vi "Double FFT Mesurament RT with Frequency Linearization & BackNoise Remove Test.vi"() -> ()   [LabVIEW 2014]
uses:
  <vilib>/Platform/TimedLoop/XDataNode/timing_clust.ctl
  <vilib>/Platform/TimedLoop/XDataNode/nitl_modes.ctl
  <vilib>/Platform/TimedLoop/XDataNode/wakeup.ctl
  <vilib>/FPGAPlugInAG/sbRIO-9636/niLvFpga_Open_sbRIO-9636.vi
  <vilib>/rvi/interface/common/dynamic/niFpgaDynamicAddResources.vi
  <vilib>/FPGAPlugInAG/Dynamic/niLvFpga_Reset_Dynamic.vi
  <vilib>/Utility/error.llb/Error Cluster From Error Code.vi
  <vilib>/rvi/errors/niLvFpgaAdjustHostInterfaceError.vi
  <vilib>/rvi/interface/common/niFpgaWaitOnOcc.vi
  <vilib>/FPGAPlugInAG/Dynamic/niLvFpga_Run_Dynamic.vi
  <vilib>/FPGAPlugInAG/Dynamic/niLvFpga_Abort_Dynamic.vi
  <vilib>/FPGAPlugInAG/Dynamic/niLvFpga_Close_Dynamic.vi
  <vilib>/rvi/interface/nirviOpenFPGA/nirviOpenFPGA.xnode
  FPGA Bitfiles/LaserDistanceSen_FPGATarget_DoubleFFTMesuram_6dDziXQAIGE.lvbitx
  FPGA Target/Test VIs/Double FFT Mesurament Test with Background Noise Remove.vi
  <vilib>/rvi/interface/nirviMethod/nirviMethod.xnode
  <vilib>/rvi/interface/nirviReadWriteControl/nirviReadWriteControl.xnode
  <vilib>/Platform/TimedLoop/XDataNode/XDataNode.xnode
  <vilib>/rvi/interface/nirviCloseFPGA/nirviCloseFPGA.xnode
  <vilib>/FPGAPlugInAG/Dynamic/niLvFpga_ConfigureFifo_Dynamic.vi
  <vilib>/rvi/errors/niLvFpgaMergeErrorWithErrorCode.vi
  <vilib>/FPGAPlugInAG/Dynamic/niLvFpga_StartFifo_Dynamic.vi
  <vilib>/rvi/interface/Simulation/niFpgaSimulationCallBeginRW.vi
  <vilib>/FPGAPlugInAG/Dynamic/niLvFpga_ReadFifo_Dynamic.vi
  <vilib>/Platform/TimedLoop/XDataNode/XDNodeRunTimeDep.lvlib
  NiFpgaLv.dll
panel:
  in  "Active PolyFit":bool
  out "2) Max-Min error":dbl
  out "1) Max-Min error":dbl
  in  "polynomial order":i32=3
  in  "side points":i32=6
  out "2^(n-bit) misure mediate":dbl
  in  "n-bit":i32=10
  in  "SubtractionType":T1(ring)=enum."LowPass"
  out "Fondo Signal":dbl[](graph)
  in  "LowPass Filter: Low cutoff frequency":dbl=1000000.0 format="%#_13g"
  in  "PolyFitting: Poly Grade":dbl=12.0
  in  "Scale Factor Rising":dbl=0.5
  out "2) Std Dev":dbl
  out "1) Std Dev":dbl
  in  "Scale Factor Falling":dbl=0.5
  in  "Triangolo dritto":bool
  in  "Acrive  Smooth":bool
  out "Complete SkewTri":dbl[](graph)
  out "2) Tri edge RISING":dbl[](graph)
  out "1) Tri edge FALLING":dbl[](graph)
  out "1) Ext Mean Time Curve":dbl[](graph)
  out "2) Ext Mean Time Curve":dbl[](graph)
  out "2) Mean Freq Curve Rising":dbl[](graph)
  out "1) Mean Freq Curve Falling":dbl[](graph)
  out "2) Freq curve":dbl[](graph)
  out "1) Freq curve":dbl[](graph)
  in  "FFT Sliding Win Size":i32=128
  out "1) SmoothSubSig":dbl[](graph)
  out "2) SmoothSubSig":dbl[](graph)
  in  "Acrive Fit":bool=TRUE
  in  "Poly Order":i32=3
  in  "Side points":i32=13
  in  "Poly Grade":dbl=5.0
  out "2) Signal&Fit 2":dbl[][](graph)
  out "1) Signal&Fit":dbl[][](graph)
  in  "tieni premuto per":i32=1
  out "Current Sig lin":i32
  in  "Acrive Linearization":bool
  in  "# Measurements for Linearization":i32=10
  in  "?":bool
  out "maxbin_secondFFT":i32
  out "maxbin_firstFFT":i32
  out "f_rise":dbl
  out "f_fall":dbl
  out "f_mean":dbl
  out "Velocity (m/s)":dbl
  out "Distance (m)":dbl
  in  "Initial Latency points":u32(slide)=400 scale=0.0..1249.0
  out "Second FFT (bin)":dbl[](graph)
  out "Second Signal (points) - Rising Triangular":dbl[](graph)
  out "First FFT (bin)":dbl[](graph)
  out "First Signal (points) - Falling Triangular":dbl[](graph)
  in  "Snapshot":bool
  in  "Windowing":T2(ring)=enum."Hanning"
  in  "first bin":i32=5
  in  "last bin":i32=255
  in  "lower limit 2":u32(slide)=738 scale=625.0..738.0
  in  "lower limit 1":u32(slide)=113 scale=0.0..113.0
  # "Estrazione del rumore di fondo (Background noise extraction)"
  # "Sav Golay Filter"
  # "WARNING:\nOnce pressed wait untill the end of operation"
  # "OFFLINE parameters"
  # "Triangolo storto\nda costante"
  # "Max Detection FFT bin range"
  # "ONLINE parameters"
  # "Se la sottrazione del fondo non è eseguita su FPGA.\n Attivarla per eseguirla lato RT"
  # "Smoothing (S-G Params)"
  # "Fitting"
  # "ONLY POWER OF 2"
  # "Min: 2 Max: 256 (2, 4, 8, 16, 32, 64, 128, 256)"
  # "LINEARIZATION FINAL RESULTS"
  # "% over Mean"
  # "%"
  # "% over Mean"
  # "%"
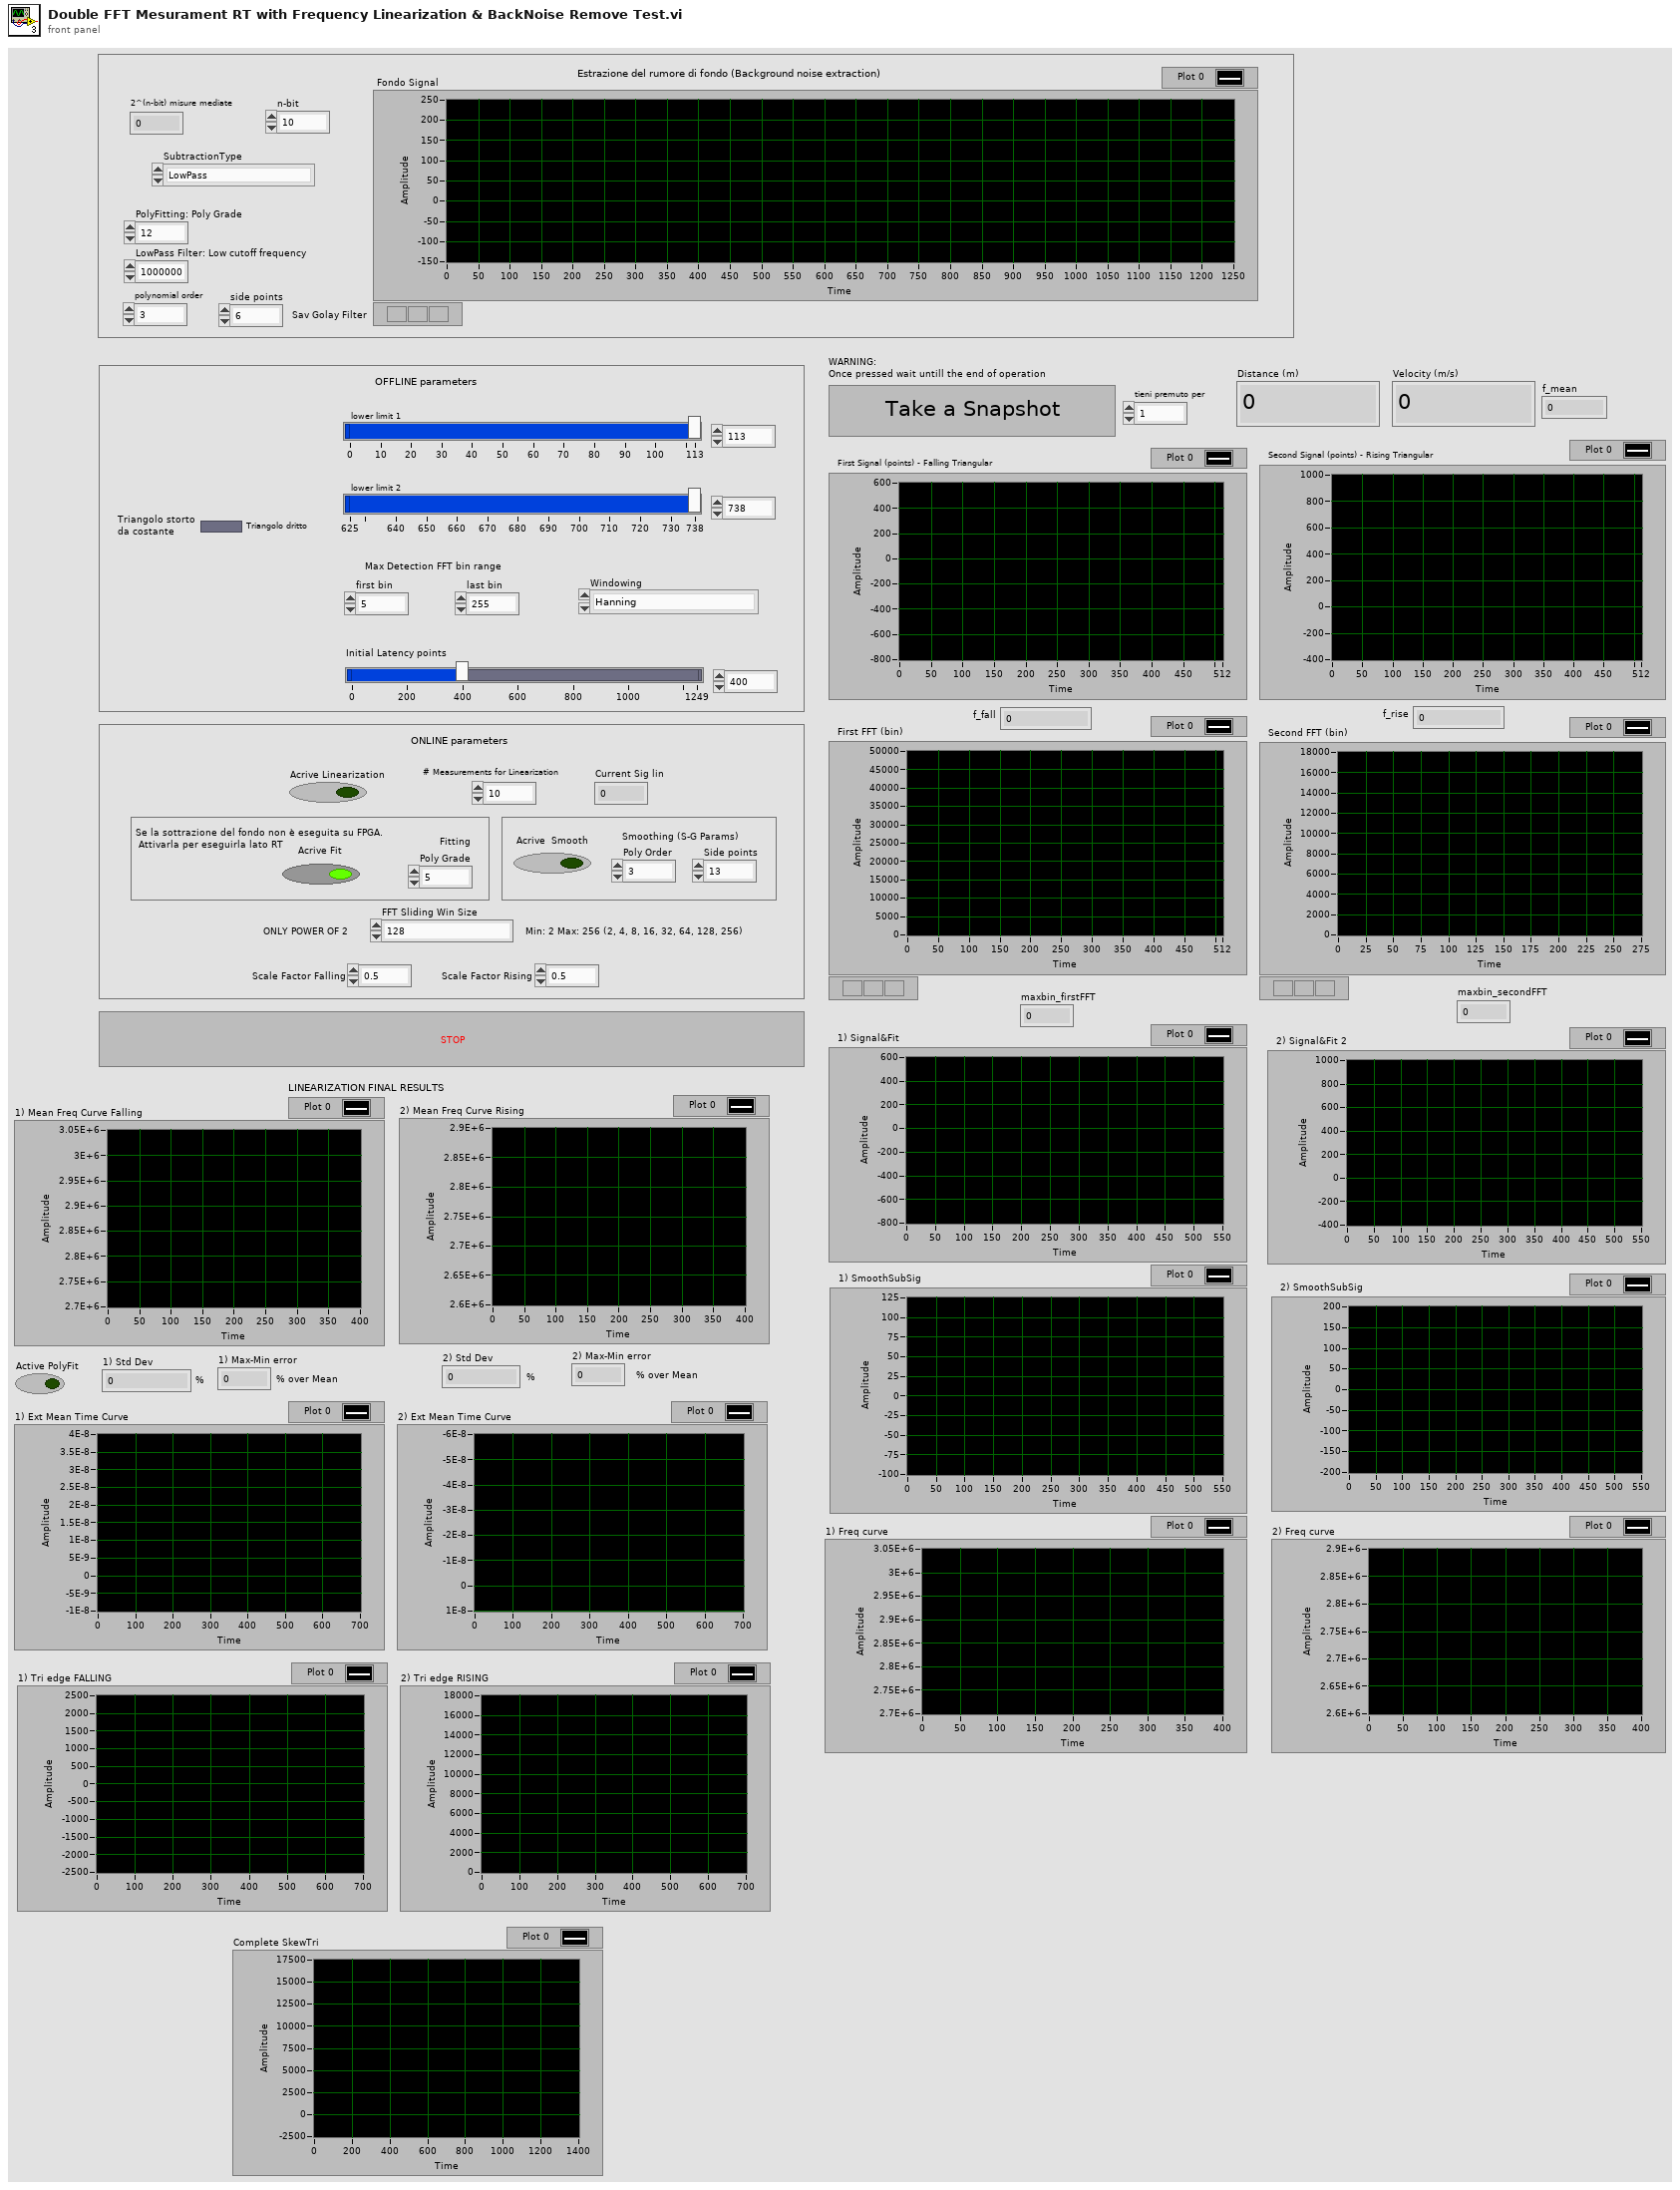
[diagram p1: front panel]
types:
  T1 = enum16{"NoSubtract", "StartingCurve", "LowPass", "PolyFitting", "SavGolay"}
  T2 = enum16{"None", "Hanning", "Hamming", "Blackman", "Blackman-Harris"}
  T3 = typedef "XDNodeRunTimeDep.lvlib/timing_clust.ctl" = cluster{"Expected End [f-1]":u64, "Actual End [f-1]":u64, "Finished Late? [f-1]":bool, "Expected End [i-1]":u64, "Actual End [i-1]":u64, "Finished Late? [i-1]":bool, "Expected Start [i]":u64, "Actual Start [i]":u64, "Expected Start [f]":u64, "Actual Start [f]":u64, "Source Name":string, "Structure Name":string, "Period":i64, "Deadline":i64, "Offset":i64, "Start":i64, "Priority":i32, "Timeout":i32, "Mode":T4, "Wakeup Reason":T5, "Error":errorcluster, "Source Type":string, "Secondary Source Type":string, "Global End Time":u64, "Global Start Time":u64, "Frame Duration":u64, "Iteration Duration":u64, "Assigned CPU":i32, "I/O Scan Engine Mode":u32}
  T4 = typedef "XDNodeRunTimeDep.lvlib/nitl_modes.ctl" = enum32{"No Change", "Process missed periods, maintain original phase", "Discard missed periods, maintain original phase", "Process missed periods, ignore original phase", "Discard missed periods, ignore original phase"}
  T5 = typedef "XDNodeRunTimeDep.lvlib/wakeup.ctl" = enum32{"Normal", "Aborted", "Asynchronous wakeup", "Timing source error", "Timed loop error", "Timeout"}
  T6 = typedef "NI_Matrix.lvlib/RealMatrix.ctl" = dbl[][]
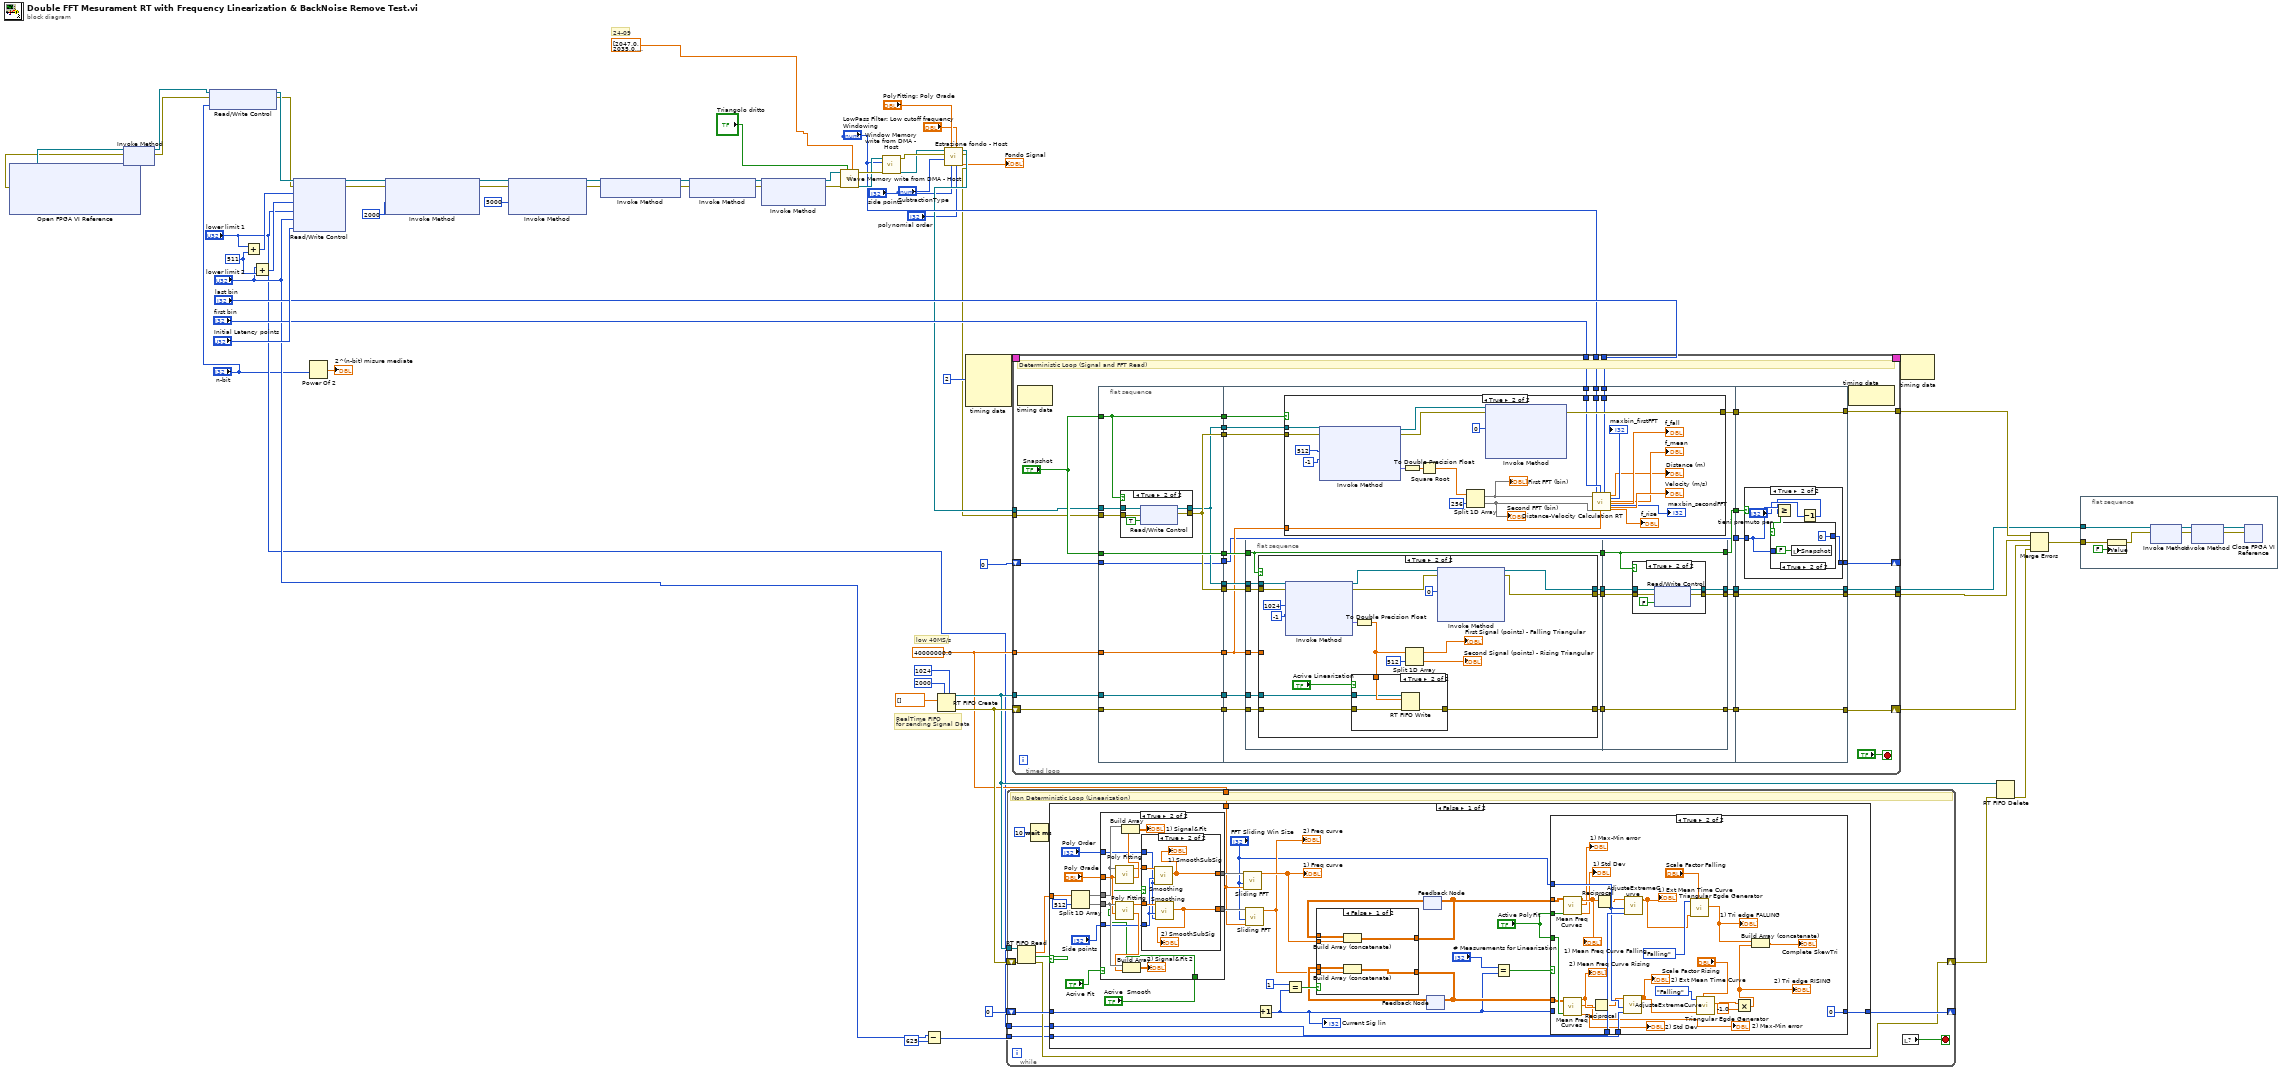
[diagram p0: block diagram]
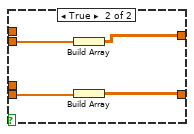
[diagram p5: hidden frame]
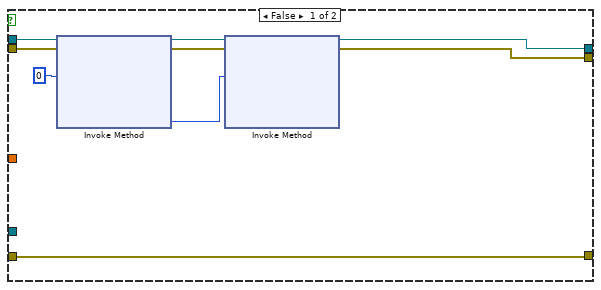
[diagram p8: hidden frame]
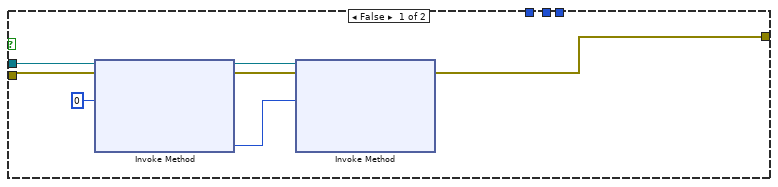
[diagram p11: hidden frame]
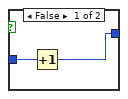
[diagram p13: hidden frame]
diagram:
  w63 = u32 511 ("y")
  w22 = 40000000.0 ("Sample Rate (S/s)")
  # "24-09"
  # "RealTime FIFO \nfor sending Signal Data"
  # "low 40MS/s"
  n1 = xnode "Open FPGA VI Reference"() -> ("FPGA VI Reference Out"=w8:refnum<k20>, "error out"=w7:errorcluster)  [unwired: 2 in]
  n2 = xnode "Invoke Method"("FPGA VI Reference In"=w8, "error in"=w7) -> ("FPGA VI Reference Out"=w5:refnum<k20>, "error out"=w3:errorcluster)
  n3 = xnode "Read/Write Control"("FPGA VI Reference In"=w5, "error in"=w3, "n-bit (2^nbit medie)"="n-bit") -> ("FPGA VI Reference Out"=w4:refnum<k20>, "error out"=w2:errorcluster)
  n4 = Add(x="lower limit 1", y=w63) -> (x+y=w65:u32)
  n5 = Add(x="lower limit 2", y=w63) -> (x+y=w64:u32)
  n6 = xnode "Read/Write Control"("FPGA VI Reference In"=w4, "error in"=w2, "upper limit 1"=w65, "upper limit 2"=w64, "lower limit 1"="lower limit 1", "lower limit 2"="lower limit 2", "Latency points"="Initial Latency points") -> ("FPGA VI Reference Out"=w62:refnum<k20>, "error out"=w61:errorcluster)
  n7 = Power Of 2(x="n-bit") -> (2^x=→"2^(n-bit) misure mediate":dbl)
  n8 = xnode "Invoke Method"("FPGA VI Reference In"=w62, "error in"=w61, "Requested Depth"=u32 2000) -> ("FPGA VI Reference Out"=w40:refnum<k20>, "error out"=w41:errorcluster)  [unwired: 1 out]
  n9 = xnode "Invoke Method"("FPGA VI Reference In"=w40, "error in"=w41, "Requested Depth"=u32 5000) -> ("FPGA VI Reference Out"=w54:refnum<k20>, "error out"=w55:errorcluster)  [unwired: 1 out]
  n10 = xnode "Invoke Method"("FPGA VI Reference In"=w54, "error in"=w55) -> ("FPGA VI Reference Out"=w38:refnum<k20>, "error out"=w39:errorcluster)
  n11 = xnode "Invoke Method"("FPGA VI Reference In"=w38, "error in"=w39) -> ("FPGA VI Reference Out"=w52:refnum<k20>, "error out"=w53:errorcluster)
  n12 = xnode "Invoke Method"("FPGA VI Reference In"=w52, "error in"=w53) -> ("FPGA VI Reference Out"=w58:refnum<k20>, "error out"=w57:errorcluster)  [unwired: 1 in]
  n13 = call "Wave Memory write from DMA - Host.vi"("Custom Triangular Signal (fal-ris)"=dbl[] [2047.0, 2035.0, 2022.0, 2010.0, 1997.0, 1985.0, 1972.0, 1960.0, 1948.0, 1935.0, 1923.0, 1911.0, 1899.0, 1886.0, 1874.0, 1862.0, 1850.0, 1838.0, 1825.0, 1813.0, 1801.0, 1789.0, 1777.0, 1765.0, 1753.0, 1741.0, 1729.0, 1717.0, 1705.0, 1693.0, 1681.0, 1669.0, 1657.0, 1645.0, 1634.0, 1622.0, 1610.0, 1598.0, 1586.0, 1575.0, 1563.0, 1551.0, 1540.0, 1528.0, 1516.0, 1505.0, 1493.0, 1481.0, 1470.0, 1458.0, 1447.0, 1435.0, 1424.0, 1412.0, 1401.0, 1389.0, 1378.0, 1366.0, 1355.0, 1344.0, 1332.0, 1321.0, 1310.0, 1298.0, 1287.0, 1276.0, 1265.0, 1253.0, 1242.0, 1231.0, 1220.0, 1209.0, 1198.0, 1186.0, 1175.0, 1164.0, 1153.0, 1142.0, 1131.0, 1120.0, 1109.0, 1098.0, 1087.0, 1076.0, 1065.0, 1055.0, 1044.0, 1033.0, 1022.0, 1011.0, 1000.0, 990.0, 979.0, 968.0, 958.0, 947.0, 936.0, 926.0, 915.0, 904.0, 894.0, 883.0, 873.0, 862.0, 852.0, 841.0, 831.0, 820.0, 810.0, 799.0, 789.0, 778.0, 768.0, 758.0, 747.0, 738.0, 727.0, 719.0, 712.0, 706.0, 700.0, 693.0, 687.0, 680.0, 674.0, 668.0, 661.0, 655.0, 648.0, 642.0, 636.0, 629.0, 623.0, 617.0, 610.0, 604.0, 598.0, 591.0, 584.0, 577.0, 569.0, 560.0, 552.0, 545.0, 538.0, 531.0, 525.0, 519.0, 512.0, 506.0, 500.0, 494.0, 488.0, 482.0, 476.0, 470.0, 464.0, 458.0, 452.0, 446.0, 436.0, 430.0, 424.0, 418.0, 412.0, 406.0, 400.0, 394.0, 388.0, 382.0, 376.0, 370.0, 364.0, 358.0, 352.0, 346.0, 338.0, 332.0, 325.0, 319.0, 313.0, 307.0, 301.0, 295.0, 290.0, 284.0, 278.0, 272.0, 267.0, 261.0, 255.0, 249.0, 244.0, 238.0, 232.0, 227.0, 221.0, 215.0, 209.0, 204.0, 198.0, 192.0, 187.0, 181.0, 175.0, 170.0, 164.0, 158.0, 153.0, 147.0, 141.0, 136.0, 130.0, 124.0, 119.0, 113.0, 108.0, 102.0, 96.0, 91.0, 85.0, 79.0, 74.0, 68.0, 62.0, 57.0, 51.0, 45.0, 39.0, 34.0, 28.0, 22.0, 16.0, 11.0, 5.0, 0.0, -6.0, -11.0, -17.0, -22.0, -28.0, -33.0, -39.0, -44.0, -50.0, -55.0, -61.0, -66.0, -72.0, -77.0, -83.0, -88.0, -94.0, -99.0, -105.0, -110.0, -116.0, -121.0, -127.0, -132.0, -137.0, -143.0, -148.0, -154.0, -159.0, -165.0, -170.0, -176.0, -181.0, -186.0, -192.0, -197.0, -203.0, -208.0, -214.0, -219.0, -224.0, -230.0, -235.0, -241.0, -246.0, -251.0, -257.0, -262.0, -268.0, -273.0, -278.0, -284.0, -289.0, -295.0, -300.0, -305.0, -311.0, -316.0, -321.0, -327.0, -332.0, -337.0, -343.0, -348.0, -354.0, -359.0, -364.0, -370.0, -375.0, -380.0, -386.0, -391.0, -397.0, -402.0, -407.0, -413.0, -418.0, -423.0, -429.0, -434.0, -439.0, -445.0, -450.0, -455.0, -461.0, -466.0, -471.0, -477.0, -482.0, -487.0, -493.0, -498.0, -503.0, -509.0, -514.0, -519.0, -525.0, -530.0, -535.0, -540.0, -546.0, -551.0, -556.0, -562.0, -567.0, -572.0, -578.0, -583.0, -588.0, -593.0, -599.0, -604.0, -609.0, -615.0, -620.0, -625.0, -630.0, -636.0, -641.0, -646.0, -651.0, -657.0, -662.0, -667.0, -673.0, -678.0, -683.0, -688.0, -694.0, -699.0, -704.0, -709.0, -715.0, -720.0, -725.0, -730.0, -736.0, -741.0, -746.0, -751.0, -757.0, -762.0, -767.0, -772.0, -778.0, -783.0, -788.0, -793.0, -799.0, -804.0, -809.0, -814.0, -820.0, -825.0, -830.0, -835.0, -841.0, -846.0, -851.0, -856.0, -862.0, -867.0, -872.0, -877.0, -883.0, -888.0, -893.0, -898.0, -903.0, -909.0, -914.0, -919.0, -924.0, -930.0, -935.0, -940.0, -945.0, -951.0, -956.0, -961.0, -966.0, -971.0, -977.0, -982.0, -987.0, -992.0, -998.0, -1003.0, -1008.0, -1013.0, -1018.0, -1024.0, -1029.0, -1034.0, -1039.0, -1045.0, -1050.0, -1055.0, -1060.0, -1065.0, -1071.0, -1076.0, -1081.0, -1086.0, -1092.0, -1097.0, -1102.0, -1107.0, -1112.0, -1118.0, -1123.0, -1128.0, -1133.0, -1138.0, -1144.0, -1149.0, -1154.0, -1159.0, -1165.0, -1170.0, -1175.0, -1180.0, -1185.0, -1191.0, -1196.0, -1201.0, -1206.0, -1211.0, -1217.0, -1222.0, -1227.0, -1232.0, -1237.0, -1243.0, -1248.0, -1253.0, -1258.0, -1263.0, -1269.0, -1274.0, -1279.0, -1284.0, -1289.0, -1295.0, -1300.0, -1305.0, -1310.0, -1315.0, -1321.0, -1326.0, -1331.0, -1336.0, -1341.0, -1347.0, -1352.0, -1357.0, -1362.0, -1367.0, -1373.0, -1378.0, -1383.0, -1388.0, -1393.0, -1399.0, -1404.0, -1409.0, -1414.0, -1419.0, -1425.0, -1430.0, -1435.0, -1440.0, -1445.0, -1450.0, -1456.0, -1461.0, -1466.0, -1471.0, -1476.0, -1482.0, -1487.0, -1492.0, -1497.0, -1502.0, -1508.0, -1513.0, -1518.0, -1523.0, -1528.0, -1534.0, -1539.0, -1544.0, -1549.0, -1554.0, -1560.0, -1565.0, -1570.0, -1575.0, -1580.0, -1586.0, -1591.0, -1596.0, -1601.0, -1606.0, -1612.0, -1617.0, -1622.0, -1627.0, -1632.0, -1637.0, -1643.0, -1648.0, -1653.0, -1658.0, -1663.0, -1669.0, -1674.0, -1679.0, -1684.0, -1689.0, -1695.0, -1700.0, -1705.0, -1710.0, -1715.0, -1721.0, -1726.0, -1731.0, -1736.0, -1741.0, -1747.0, -1752.0, -1757.0, -1762.0, -1767.0, -1773.0, -1778.0, -1783.0, -1788.0, -1793.0, -1799.0, -1804.0, -1809.0, -1814.0, -1819.0, -1825.0, -1830.0, -1835.0, -1840.0, -1845.0, -1851.0, -1856.0, -1861.0, -1866.0, -1871.0, -1876.0, -1882.0, -1887.0, -1892.0, -1897.0, -1902.0, -1908.0, -1913.0, -1918.0, -1923.0, -1928.0, -1934.0, -1939.0, -1944.0, -1949.0, -1954.0, -1960.0, -1965.0, -1970.0, -1975.0, -1980.0, -1986.0, -1991.0, -1996.0, -2001.0, -2006.0, -2012.0, -2017.0, -2022.0, -2027.0, -2032.0, -2038.0, -2043.0, -2048.0, -2047.0, -2037.0, -2027.0, -2017.0, -2007.0, -1997.0, -1987.0, -1977.0, -1967.0, -1957.0, -1947.0, -1937.0, -1927.0, -1917.0, -1907.0, -1897.0, -1888.0, -1878.0, -1868.0, -1858.0, -1848.0, -1838.0, -1828.0, -1819.0, -1809.0, -1799.0, -1789.0, -1780.0, -1770.0, -1760.0, -1750.0, -1741.0, -1731.0, -1721.0, -1712.0, -1702.0, -1692.0, -1683.0, -1673.0, -1663.0, -1654.0, -1644.0, -1635.0, -1625.0, -1615.0, -1606.0, -1596.0, -1587.0, -1577.0, -1568.0, -1558.0, -1549.0, -1539.0, -1530.0, -1520.0, -1511.0, -1501.0, -1492.0, -1483.0, -1473.0, -1464.0, -1454.0, -1445.0, -1436.0, -1426.0, -1417.0, -1408.0, -1398.0, -1389.0, -1380.0, -1371.0, -1361.0, -1352.0, -1343.0, -1334.0, -1324.0, -1315.0, -1306.0, -1297.0, -1288.0, -1278.0, -1269.0, -1260.0, -1251.0, -1242.0, -1233.0, -1224.0, -1215.0, -1205.0, -1196.0, -1187.0, -1178.0, -1169.0, -1160.0, -1151.0, -1142.0, -1133.0, -1124.0, -1115.0, -1106.0, -1097.0, -1088.0, -1080.0, -1071.0, -1062.0, -1053.0, -1044.0, -1035.0, -1026.0, -1017.0, -1009.0, -1000.0, -991.0, -982.0, -973.0, -965.0, -953.0, -944.0, -935.0, -920.0, -906.0, -889.0, -871.0, -854.0, -842.0, -834.0, -826.0, -818.0, -810.0, -802.0, -794.0, -786.0, -778.0, -770.0, -762.0, -754.0, -746.0, -739.0, -731.0, -723.0, -715.0, -707.0, -699.0, -690.0, -682.0, -672.0, -661.0, -651.0, -639.0, -627.0, -616.0, -606.0, -598.0, -591.0, -584.0, -577.0, -570.0, -563.0, -556.0, -549.0, -542.0, -535.0, -528.0, -520.0, -513.0, -506.0, -499.0, -492.0, -485.0, -478.0, -471.0, -464.0, -457.0, -451.0, -444.0, -437.0, -430.0, -423.0, -416.0, -409.0, -400.0, -390.0, -382.0, -373.0, -364.0, -356.0, -349.0, -343.0, -336.0, -330.0, -323.0, -317.0, -310.0, -304.0, -297.0, -291.0, -284.0, -278.0, -271.0, -265.0, -258.0, -252.0, -245.0, -239.0, -232.0, -226.0, -219.0, -213.0, -207.0, -200.0, -194.0, -187.0, -181.0, -175.0, -168.0, -162.0, -156.0, -149.0, -143.0, -136.0, -128.0, -121.0, -114.0, -107.0, -100.0, -93.0, -87.0, -80.0, -74.0, -68.0, -62.0, -56.0, -50.0, -44.0, -38.0, -32.0, -26.0, -20.0, -14.0, -8.0, -2.0, 5.0, 11.0, 17.0, 23.0, 29.0, 35.0, 41.0, 47.0, 53.0, 59.0, 65.0, 70.0, 76.0, 82.0, 88.0, 94.0, 100.0, 106.0, 112.0, 118.0, 124.0, 130.0, 136.0, 142.0, 148.0, 154.0, 161.0, 167.0, 174.0, 180.0, 186.0, 192.0, 198.0, 204.0, 210.0, 215.0, 221.0, 227.0, 233.0, 238.0, 244.0, 250.0, 255.0, 261.0, 267.0, 273.0, 278.0, 284.0, 290.0, 295.0, 301.0, 307.0, 312.0, 318.0, 324.0, 329.0, 335.0, 341.0, 346.0, 352.0, 358.0, 363.0, 369.0, 374.0, 380.0, 386.0, 391.0, 397.0, 402.0, 408.0, 414.0, 419.0, 425.0, 430.0, 436.0, 441.0, 447.0, 453.0, 458.0, 464.0, 470.0, 475.0, 481.0, 487.0, 493.0, 499.0, 504.0, 510.0, 516.0, 521.0, 527.0, 532.0, 538.0, 543.0, 549.0, 554.0, 560.0, 565.0, 571.0, 576.0, 582.0, 587.0, 593.0, 598.0, 604.0, 609.0, 614.0, 620.0, 625.0, 631.0, 636.0, 642.0, 647.0, 653.0, 658.0, 663.0, 669.0, 674.0, 680.0, 685.0, 691.0, 696.0, 701.0, 707.0, 712.0, 718.0, 723.0, 728.0, 734.0, 739.0, 745.0, 750.0, 755.0, 761.0, 766.0, 772.0, 777.0, 782.0, 788.0, 793.0, 798.0, 804.0, 809.0, 815.0, 820.0, 826.0, 831.0, 837.0, 842.0, 847.0, 853.0, 858.0, 863.0, 869.0, 874.0, 880.0, 885.0, 890.0, 895.0, 901.0, 906.0, 911.0, 917.0, 922.0, 927.0, 933.0, 938.0, 943.0, 948.0, 954.0, 959.0, 964.0, 970.0, 975.0, 980.0, 985.0, 991.0, 996.0, 1001.0, 1006.0, 1012.0, 1017.0, 1022.0, 1027.0, 1033.0, 1038.0, 1043.0, 1048.0, 1054.0, 1059.0, 1064.0, 1069.0, 1075.0, 1080.0, 1085.0, 1090.0, 1096.0, 1101.0, 1106.0, 1111.0, 1116.0, 1122.0, 1127.0, 1132.0, 1137.0, 1143.0, 1148.0, 1153.0, 1158.0, 1163.0, 1169.0, 1174.0, 1179.0, 1184.0, 1190.0, 1195.0, 1200.0, 1205.0, 1211.0, 1216.0, 1221.0, 1226.0, 1231.0, 1237.0, 1242.0, 1247.0, 1252.0, 1257.0, 1262.0, 1268.0, 1273.0, 1278.0, 1283.0, 1288.0, 1293.0, 1298.0, 1304.0, 1309.0, 1314.0, 1319.0, 1324.0, 1329.0, 1334.0, 1340.0, 1345.0, 1350.0, 1355.0, 1360.0, 1365.0, 1370.0, 1375.0, 1381.0, 1386.0, 1391.0, 1396.0, 1401.0, 1406.0, 1411.0, 1416.0, 1421.0, 1427.0, 1432.0, 1437.0, 1442.0, 1447.0, 1452.0, 1457.0, 1462.0, 1467.0, 1472.0, 1478.0, 1483.0, 1488.0, 1493.0, 1498.0, 1503.0, 1508.0, 1513.0, 1518.0, 1523.0, 1528.0, 1534.0, 1539.0, 1544.0, 1549.0, 1554.0, 1559.0, 1564.0, 1569.0, 1574.0, 1579.0, 1584.0, 1589.0, 1595.0, 1600.0, 1605.0, 1610.0, 1615.0, 1620.0, 1625.0, 1630.0, 1635.0, 1640.0, 1645.0, 1650.0, 1655.0, 1660.0, 1666.0, 1671.0, 1676.0, 1681.0, 1686.0, 1691.0, 1696.0, 1701.0, 1706.0, 1711.0, 1716.0, 1721.0, 1726.0, 1731.0, 1736.0, 1741.0, 1746.0, 1751.0, 1757.0, 1762.0, 1767.0, 1772.0, 1777.0, 1782.0, 1787.0, 1792.0, 1797.0, 1802.0, 1807.0, 1812.0, 1817.0, 1822.0, 1827.0, 1832.0, 1837.0, 1842.0, 1847.0, 1852.0, 1857.0, 1862.0, 1867.0, 1872.0, 1877.0, 1883.0, 1888.0, 1893.0, 1898.0, 1903.0, 1908.0, 1913.0, 1918.0, 1923.0, 1928.0, 1933.0, 1938.0, 1943.0, 1948.0, 1953.0, 1958.0, 1963.0, 1968.0, 1973.0, 1978.0, 1983.0, 1988.0, 1993.0, 1998.0, 2003.0, 2008.0, 2013.0, 2018.0, 2023.0, 2028.0, 2033.0, 2038.0, 2043.0, 2048.0] ("appended array"), "Triangolo dritto?"="Triangolo dritto", "error in"=w57, "FPGA VI Reference In"=w58) -> ("FPGA VI Reference Out"=w43:refnum<k20>, "error out"=w56:errorcluster)  [unwired: 5 in, 1 out]
  n14 = call "Window Memory write from DMA - Host.vi"("error in"=w56, "Enum"="Windowing", "FPGA VI Reference In"=w43) -> ("FPGA VI Reference Out"=w18:refnum<k20>, "error out"=w19:errorcluster)  [unwired: 5 in, 2 out]
  n15 = Subtract(x="lower limit 2", y=u32 625) -> (x-y=w24:u32)
  n16 = RT FIFO Create(1:dbl[] [] ("double precision float"), 4:u32 2000 ("size (10)"), 6:u32 1024 ("elements in array (1)")) -> (8:w30:refnum<k33>, 11:w32:errorcluster)  [unwired: 5 in, 1 out]
  n17 = call "Estrazione fondo - Host.vi"("polynomial order"="polynomial order", "LowPass Filter: Low cutoff frequency"="LowPass Filter: Low cutoff frequency", "side points"="side points", "PolyFitting: Poly Grade"="PolyFitting: Poly Grade", "SubtractionType"="SubtractionType", "error in"=w19, "FPGA VI Reference In"=w18) -> ("Fondo Signal"=→"Fondo Signal":dbl[], "error out"=w16:errorcluster, "FPGA VI Reference Out"=w17:refnum<k20>)  [unwired: 1 in, 1 out]
  n18 = node-c288(i64 2 ("Period")) -> (w51:T3)  [unwired: 3 in]
  n19 = while {
    shift-right: [w69] -> w29
    shift-left: w32 -> [w71]
    tunnel: w30 -> [w76]
    shift-right: [w70] -> _
    shift-left: 0 -> [w74]
    tunnel: "lower limit 1" -> [w66]
    tunnel: w24 -> [w67]
    tunnel: w22 -> [w68]
    stop <- w75 stop-if-true
    # "Non Deterministic Loop (Linearization)"
    n20 = RT FIFO Read(0:w76, 3:w71) -> (9:w73:dbl[], 10:w72:bool, 11:w69:errorcluster)  [unwired: 2 in, 2 out]
    n21 = Wait (ms)(milliseconds to wait=u32 10 ("millisecond multiple")) -> ()  [unwired: 1 out]
    n22 = case shown="False" w72 {
      tunnel: w74 -> [w106 w169]
      tunnel: [w95 w169] -> w70
      tunnel: w73 -> [w104 _]
      tunnel: w68 -> [w85 _]
      tunnel: w67 -> [w82 _]
      tunnel: w66 -> [w81 _]
      frame False {
        n23 = Split 1D Array(array=w104, index=512) -> (first subarray=w93:dbl[], second subarray=w92:dbl[])
        n24 = case shown="True" "Acrive Fit" {
          tunnel: w93 -> [w108 w122]
          tunnel: w92 -> [w107 w118]
          tunnel: "Poly Grade" -> [_ w114]
          tunnel: "Side points" -> [_ w113]
          tunnel: "Poly Order" -> [_ w112]
          tunnel: [w107 w111] -> w86
          tunnel: [w108 w109] -> w87
          tunnel: "Acrive  Smooth" -> [_ w110]
          frame False {
          }
          frame True {
            n25 = call "Poly Fitting.vi"("Poly Grade"=w114, "Signal"=w122) -> ("Poly Signal"=w121:dbl[], "SubtractedSignal"=w116:dbl[])  [unwired: 8 in]
            n26 = call "Poly Fitting.vi"("Poly Grade"=w114, "Signal"=w118) -> ("Poly Signal"=w117:dbl[], "SubtractedSignal"=w115:dbl[])  [unwired: 8 in]
            n27 = Build Array(w122, w121) -> (→"1) Signal&Fit":dbl[][])
            n28 = Build Array(w118, w117) -> (→"2) Signal&Fit 2":dbl[][])
            n29 = case shown="True" w110 {
              tunnel: w116 -> [w124 w130]
              tunnel: w115 -> [w123 w129]
              tunnel: w113 -> [_ w128]
              tunnel: w112 -> [_ w127]
              tunnel: [w123 w126] -> w111
              tunnel: [w124 w125] -> w109
              frame False {
              }
              frame True {
                n30 = call "Smoothing.vi"("polynomial order"=w127, "side points"=w128, "SubtractedSignal"=w130) -> ("SubSmoothSignal"=w125:dbl[])  [unwired: 8 in]
                "1) SmoothSubSig" <- w125
                n31 = call "Smoothing.vi"("polynomial order"=w127, "side points"=w128, "SubtractedSignal"=w129) -> ("SubSmoothSignal"=w126:dbl[])  [unwired: 8 in]
                "2) SmoothSubSig" <- w126
              }
            }
          }
        }
        n32 = call "Sliding FFT.vi"("Sample Freq"=w85, "FFT Win Size"="FFT Sliding Win Size", "SubSmoothSignal"=w87) -> ("Freq samples"=w84:dbl[])  [unwired: 7 in, 1 out]
        "1) Freq curve" <- w84
        n33 = call "Sliding FFT.vi"("Sample Freq"=w85, "FFT Win Size"="FFT Sliding Win Size", "SubSmoothSignal"=w86) -> ("Freq samples"=w83:dbl[])  [unwired: 7 in, 1 out]
        "2) Freq curve" <- w83
        n34 = Increment(x=w106) -> (x+1=w96:i32)
        "Current Sig lin" <- w96
        n35 = Equal?(x=1, y=w96) -> (x = y?=w102:bool)
        n36 = feedback #1() -> (w101:T6)  [unwired: 1 in]
        n37 = feedback #2() -> (w100:T6)  [unwired: 1 in]
        n38 = case shown="False" w102 {
          tunnel: w83 -> [w163 w166]
          tunnel: w84 -> [w164 w168]
          tunnel: [w162 w165] -> w97
          tunnel: [w161 w167] -> w98
          tunnel: w101 -> [w160 _]
          tunnel: w100 -> [w159 _]
          frame False {
            n39 = Build Array (concatenate)(w160, w164) -> (w161:T6)
            n40 = Build Array (concatenate)(w159, w163) -> (w162:T6)
          }
          frame True {
            n41 = Build Array(w168) -> (w167:T6)
            n42 = Build Array(w166) -> (w165:T6)
          }
        }
        n43 = feedback-in #1(w98) -> ()
        n44 = feedback-in #2(w97) -> ()
        n45 = Equal?(x="# Measurements for Linearization", y=w96) -> (x = y?=w94:bool)
        n46 = case shown="True" w94 {
          tunnel: w98 -> [_ w141]
          tunnel: w97 -> [_ w132]
          tunnel: w96 -> [w131 _]
          tunnel: [w131 0] -> w95
          tunnel: w82 -> [_ w153]
          tunnel: w81 -> [_ w152]
          tunnel: "FFT Sliding Win Size" -> [_ w151]
          tunnel: "Active PolyFit" -> [_ w134]
          tunnel: "Active PolyFit" -> [_ w133]
          frame False {
          }
          frame True {
            n47 = call "Mean Freq Curves.vi"("Set of Freq samples"=w141, "Active Fit"=w134) -> ("Mean Freq Curve"=w140:dbl[], "Max-Min error (% over Mean)"=→"1) Max-Min error":dbl, "StdDev%"=→"1) Std Dev":dbl)  [unwired: 12 in, 3 out]
            "1) Mean Freq Curve Falling" <- w140
            n48 = call "Mean Freq Curves.vi"("Set of Freq samples"=w132, "Active Fit"=w133) -> ("Mean Freq Curve"=w137:dbl[], "Max-Min error (% over Mean)"=→"2) Max-Min error":dbl, "StdDev%"=→"2) Std Dev":dbl)  [unwired: 12 in, 3 out]
            "2) Mean Freq Curve Rising" <- w137
            n49 = Reciprocal(x=w137) -> (1/x=w148:dbl[])
            n50 = Reciprocal(x=w140) -> (1/x=w147:dbl[])
            n51 = call "AdjusteExtremeCurve.vi"("Init Bins Discarded"=w153, "FFT Size Window"=w151, "Freq sample"=w148) -> ("Extended Freq Sample"=w149:dbl[])  [unwired: 8 in]
            "2) Ext Mean Time Curve" <- w149
            n52 = call "AdjusteExtremeCurve.vi"("Init Bins Discarded"=w152, "FFT Size Window"=w151, "Freq sample"=w147) -> ("Extended Freq Sample"=w150:dbl[])  [unwired: 8 in]
            "1) Ext Mean Time Curve" <- w150
            n53 = call "Triangular Egde Generator.vi"("fattore"="Scale Factor Falling", "Sample values"=w150, "Triangular edge"=enum16{"Rising", "Falling"}."Falling") -> ("Skew Triangular"=w155:dbl[])  [unwired: 8 in]
            "1) Tri edge FALLING" <- w155
            n54 = call "Triangular Egde Generator.vi"("fattore"="Scale Factor Rising", "Sample values"=w149, "Triangular edge"=enum16{"Rising", "Falling"}."Falling") -> ("Skew Triangular"=w145:dbl[])  [unwired: 8 in]
            n55 = Multiply(x=w145, y=-1.0) -> (x*y=w144:dbl[])
            "2) Tri edge RISING" <- w144
            n56 = Build Array (concatenate)(w155, w144) -> (→"Complete SkewTri":dbl[])
          }
        }
      }
      frame True {
      }
    }
    n57 = local read item#18() -> (w75:bool)
  }
  n58 = timed-loop {
    tunnel: w17 -> [w196]
    tunnel: w16 -> [w197]
    tunnel: [w199] -> w48
    tunnel: w22 -> [w201]
    tunnel: [w200] -> w47
    timing: w51 -> [_]
    timing-out: [_] -> w50
    tunnel: "first bin" -> [w185]
    tunnel: "last bin" -> [w184]
    tunnel: [w182] -> w42
    tunnel: "Windowing" -> [w180]
    shift-right: [w174] -> w33
    shift-left: w32 -> [w176]
    tunnel: w30 -> [w178]
    shift-right: [w170] -> _
    shift-left: 0 -> [w172]
    stop <- "?" stop-if-true
    # "Deterministic Loop (Signal and FFT Read)"
    n59 = node-c288() -> ()  [unwired: 1 in, 1 out]
    n60 = flat-sequence {
      tunnel: w196 -> [w209]
      tunnel: w197 -> [w210]
      tunnel: "Snapshot" -> [w207]
      tunnel: "Snapshot" -> [w212]
      tunnel: w201 -> [w213]
      tunnel: [w211] -> w195
      tunnel: [w213] -> w194
      tunnel: [w212] -> w193
      tunnel: [w207] -> w192
      tunnel: [w211] -> w191
      tunnel: [w208] -> w190
      tunnel: [w208] -> w189
      tunnel: [w206] -> w179
      tunnel: w178 -> [w206]
      tunnel: [w205] -> w177
      tunnel: w176 -> [w205]
      tunnel: [w204] -> w173
      tunnel: w172 -> [w204]
      tunnel: w195 -> [w238]
      tunnel: w194 -> [w226]
      tunnel: w193 -> [w232]
      tunnel: w192 -> [w235]
      tunnel: w191 -> [w234]
      tunnel: w190 -> [w233]
      tunnel: w189 -> [w239]
      tunnel: [w237] -> w188
      tunnel: [w236] -> w187
      tunnel: [w231] -> w186
      tunnel: w185 -> [w230]
      tunnel: w184 -> [w229]
      tunnel: [w228] -> w181
      tunnel: w180 -> [w227]
      tunnel: w179 -> [w225]
      tunnel: w177 -> [w224]
      tunnel: [w222] -> w175
      tunnel: w173 -> [w221]
      tunnel: [w221] -> w171
      tunnel: [w334] -> w199
      tunnel: [w335] -> w200
      tunnel: w188 -> [w335]
      tunnel: w187 -> [w334]
      tunnel: w186 -> [w333]
      tunnel: [w332] -> w182
      tunnel: w181 -> [w332]
      tunnel: [w331] -> w174
      tunnel: w175 -> [w331]
      tunnel: w171 -> [w330]
      tunnel: [w329] -> w170
      frame #0 {
        n61 = case shown="True" w207 {
          tunnel: [w214 w219] -> w211
          tunnel: w210 -> [w214 w218]
          tunnel: w209 -> [w215 w217]
          tunnel: [w215 w216] -> w208
          frame False {
          }
          frame True {
            n62 = xnode "Read/Write Control"("FPGA VI Reference In"=w217, "error in"=w218, "snapshot"=TRUE) -> ("FPGA VI Reference Out"=w216:refnum<k20>, "error out"=w219:errorcluster)
          }
        }
      }
      frame #1 {
        n63 = flat-sequence {
          tunnel: w239 -> [w251]
          tunnel: w238 -> [w250]
          tunnel: w226 -> [w249]
          tunnel: w232 -> [w246]
          tunnel: [w248] -> w242
          tunnel: [w247] -> w241
          tunnel: [w246] -> w240
          tunnel: w225 -> [w245]
          tunnel: w224 -> [w244]
          tunnel: [w243] -> w223
          tunnel: [w287] -> w236
          tunnel: w242 -> [w289]
          tunnel: w241 -> [w288]
          tunnel: w240 -> [w286]
          tunnel: [w286] -> w231
          tunnel: [w285] -> w228
          tunnel: [w284] -> w222
          tunnel: w223 -> [w284]
          frame #0 {
            n64 = case shown="True" w246 {
              tunnel: w251 -> [w259 w278]
              tunnel: w250 -> [w257 w277]
              tunnel: [w256 w270] -> w247
              tunnel: w249 -> [_ _]
              tunnel: [w253 w269] -> w248
              tunnel: w245 -> [_ w264]
              tunnel: w244 -> [w252 w263]
              tunnel: [w252 w262] -> w243
              frame False {
                n65 = xnode "Invoke Method"("FPGA VI Reference In"=w259, "error in"=w257, "Number of Elements"=u32 0) -> ("FPGA VI Reference Out"=w255:refnum<k20>, "error out"=w254:errorcluster, "Elements Remaining"=w258:u32)  [unwired: 1 in, 1 out]
                n66 = xnode "Invoke Method"("FPGA VI Reference In"=w255, "error in"=w254, "Number of Elements"=w258) -> ("FPGA VI Reference Out"=w253:refnum<k20>, "error out"=w256:errorcluster)  [unwired: 1 in, 2 out]
              }
              frame True {
                n67 = xnode "Invoke Method"("FPGA VI Reference In"=w278, "error in"=w277, "Number of Elements"=u32 1024, "Timeout (ms)"=-1) -> ("FPGA VI Reference Out"=w272:refnum<k20>, "error out"=w271:errorcluster, "Data"=w274:fxp<+/-,12,12>[])  [unwired: 1 out]
                n68 = To Double Precision Float(number=w274) -> (double precision float=w265:dbl[])
                n69 = case shown="True" "Acrive Linearization" {
                  tunnel: w265 -> [_ w283]
                  tunnel: w264 -> [_ w282]
                  tunnel: w263 -> [w279 w281]
                  tunnel: [w279 w280] -> w262
                  frame False {
                  }
                  frame True {
                    n70 = RT FIFO Write(0:w282, 1:w283, 3:w281) -> (11:w280:errorcluster)  [unwired: 2 in, 3 out]
                  }
                }
                n71 = Split 1D Array(array=w265, index=512) -> (first subarray=→"First Signal (points) - Falling Triangular":dbl[], second subarray=→"Second Signal (points) - Rising Triangular":dbl[])
                n72 = xnode "Invoke Method"("FPGA VI Reference In"=w272, "error in"=w271, "Number of Elements"=u32 0) -> ("FPGA VI Reference Out"=w269:refnum<k20>, "error out"=w270:errorcluster)  [unwired: 1 in, 2 out]
              }
            }
          }
          frame #1 {
            n73 = case shown="True" w286 {
              tunnel: [w291 w294] -> w287
              tunnel: w289 -> [w290 w295]
              tunnel: w288 -> [w291 w293]
              tunnel: [w290 w292] -> w285
              frame False {
              }
              frame True {
                n74 = xnode "Read/Write Control"("FPGA VI Reference In"=w295, "error in"=w293, "snapshot"=FALSE) -> ("FPGA VI Reference Out"=w292:refnum<k20>, "error out"=w294:errorcluster)
              }
            }
          }
        }
        n75 = case shown="True" w235 {
          tunnel: w233 -> [w302 w323]
          tunnel: w234 -> [w299 w324]
          tunnel: [w298 w322] -> w237
          tunnel: w230 -> [_ w309]
          tunnel: w229 -> [_ w310]
          tunnel: w227 -> [_ w306]
          tunnel: w226 -> [_ w304]
          frame False {
            n76 = xnode "Invoke Method"("FPGA VI Reference In"=w302, "error in"=w299, "Number of Elements"=u32 0) -> ("FPGA VI Reference Out"=w300:refnum<k20>, "error out"=w297:errorcluster, "Elements Remaining"=w301:u32)  [unwired: 1 in, 1 out]
            n77 = xnode "Invoke Method"("FPGA VI Reference In"=w300, "error in"=w297, "Number of Elements"=w301) -> ("error out"=w298:errorcluster)  [unwired: 1 in, 3 out]
          }
          frame True {
            n78 = xnode "Invoke Method"("FPGA VI Reference In"=w323, "error in"=w324, "Number of Elements"=u32 512, "Timeout (ms)"=-1) -> ("FPGA VI Reference Out"=w320:refnum<k20>, "error out"=w321:errorcluster, "Data"=w326:fxp<+,44,44>[])  [unwired: 1 out]
            n79 = To Double Precision Float(number=w326) -> (double precision float=w325:dbl[])
            n80 = Square Root(x=w325) -> (sqrt(x)=w318:dbl[])
            n81 = Split 1D Array(array=w318, index=256) -> (first subarray=w316:dbl[], second subarray=w315:dbl[])
            "First FFT (bin)" <- w316
            "Second FFT (bin)" <- w315
            n82 = xnode "Invoke Method"("FPGA VI Reference In"=w320, "error in"=w321, "Number of Elements"=u32 0) -> ("error out"=w322:errorcluster)  [unwired: 1 in, 3 out]
            n83 = call "Distance-Velocity Calculation RT.vi"("First FFT"=w316, "Second FFT"=w315, "Windowing"=w306, "first FFT bin"=w309, "Sample Rate (S/s)"=w304, "last FFT bin"=w310) -> ("F_rise"=→"f_rise":dbl, "maxbin_firstFFT"=→"maxbin_firstFFT":i32, "maxbin_secondFFT"=→"maxbin_secondFFT":i32, "Distance (m)"=→"Distance (m)":dbl, "f_mean"=→"f_mean":dbl, "F_fall"=→"f_fall":dbl, "Velocity (m/s)"=→"Velocity (m/s)":dbl)  [unwired: 7 in]
          }
        }
      }
      frame #2 {
        n84 = case shown="True" w333 {
          tunnel: w330 -> [w336 w340]
          tunnel: [w336 w341] -> w329
          frame False {
          }
          frame True {
            n85 = Decrement(x="tieni premuto per") -> (x-1=w337:i32)
            n86 = Greater Or Equal?(x=w340, y=w337) -> (x >= y?=w339:bool)
            n87 = case shown="True" w339 {
              tunnel: w340 -> [w342 _]
              tunnel: [w343 0] -> w341
              frame False {
                n88 = Increment(x=w342) -> (x+1=w343:i32)
              }
              frame True {
                n89 = local write "Snapshot"(FALSE ("Snapshot")) -> ()
              }
            }
          }
        }
      }
    }
    n90 = node-c288() -> ()  [unwired: 1 in, 1 out]
  }
  n91 = node-c288(w50) -> ()  [unwired: 1 out]
  n92 = RT FIFO Delete(0:w30, 3:w29) -> (11:w28:errorcluster)  [unwired: 1 in]
  n93 = Merge Errors(w47, w48, w33, w28) -> (w31:errorcluster)
  n94 = flat-sequence {
    tunnel: w31 -> [w349]
    tunnel: w42 -> [w346]
    frame #0 {
      n95 = property class="Bool (strict)"(error in=w349, "Value"=FALSE ("stop")) -> (error out=w348:errorcluster)  [unwired: 1 in, 1 out]
      n96 = xnode "Invoke Method"("FPGA VI Reference In"=w346, "error in"=w348) -> ("FPGA VI Reference Out"=w351:refnum<k20>, "error out"=w350:errorcluster)
      n97 = xnode "Invoke Method"("FPGA VI Reference In"=w351, "error in"=w350) -> ("FPGA VI Reference Out"=w352:refnum<k20>, "error out"=w353:errorcluster)
      n98 = xnode "Close FPGA VI Reference"("FPGA VI Reference In"=w352, "error in"=w353) -> ()  [unwired: 1 out]
    }
  }
